vi "IR Transmit NEC.vi"(8 "Error In":errorcluster, 9 "Data":u8=52, 10 "Address":u8=52, 11 "Arduino Resource":T1={"VISA resource"="", "Board Type"=enum."Uno", "Connection Type"=enum."USB / Serial", "Bytes Per Packet (15)"=15}) -> (0 "Error Out":errorcluster, 3 "Arduino Resource":T1={"VISA resource"="", "Board Type"=enum."Uno", "Connection Type"=enum."USB / Serial", "Bytes Per Packet (15)"=15})   [LabVIEW 2015, in "LabVIEW Interface for Arduino.lvlib"]
uses:
  <vilib>/LabVIEW Interface for Arduino/LabVIEW Interface for Arduino.lvlib
  <vilib>/LabVIEW Interface for Arduino/Type Defs/Arduino Resource.ctl
  <vilib>/LabVIEW Interface for Arduino/Type Defs/Board Type.ctl
  <vilib>/LabVIEW Interface for Arduino/Type Defs/IR Type.ctl
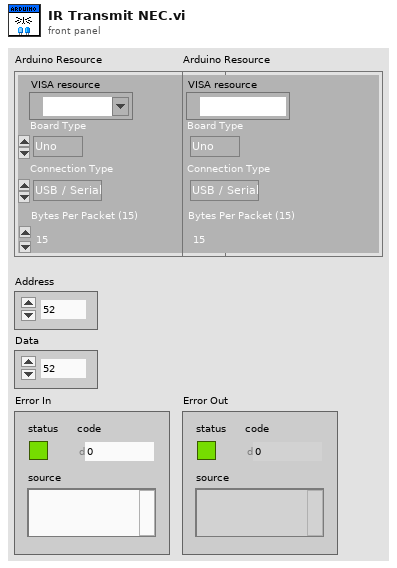
[diagram p1: front panel]
types:
  T1 = typedef "LabVIEW Interface for Arduino.lvlib/Arduino Resource.ctl" = cluster{"VISA resource":refnum<visa-resource-name>, "Board Type":T2, "Connection Type":enum8{"USB / Serial"}, "Bytes Per Packet (15)":u8}
  T2 = typedef "LabVIEW Interface for Arduino.lvlib/Board Type.ctl" = enum16{"Uno", "Dimuelanove w/Atmega 328", "Mega 2560"}
  T3 = typedef "IR Type.ctl" = enum8{"NEC", "Sony", "RC5", "RC6"}
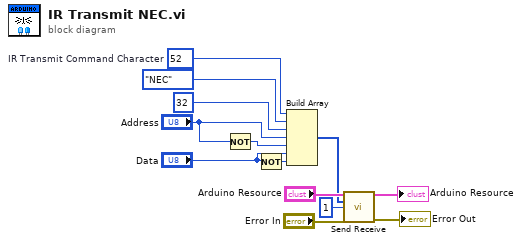
[diagram p0: block diagram]
diagram:
  w2 = u8 52  # IR Transmit Command Character
  n1 = Not(x="Address") -> (.not. x?=w5:u8)
  n2 = Not(x="Data") -> (.not. x?=w3:u8)
  n3 = Build Array(w2, IR_Type."NEC" ("IR Type"), u8 32 ("element"), "Address", w5, "Data", w3) -> (w9:u8[])
  n4 = call <vilib>:"Send Receive.vi"("Arduino Resource"="Arduino Resource", "Data"=w9, "Bytes To Read (0)"=u32 1, "error in"="Error In") -> ("Arduino Resource"=→"Arduino Resource":T1, "error out"=→"Error Out":errorcluster)  [unwired: 9 in, 1 out]
